vi "TestExec.Result Option, Level to Control.vi"(10 "Level":i32) -> (2 "Result Sel Out":T1=1 items=["Enabled", "Disabled"])   [LabVIEW 2018]
uses:
  TestExec.Result Option Selector.ctl
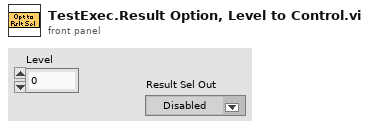
[diagram p1: front panel]
types:
  T1 = typedef "TestExec.Result Option Selector.ctl" = u16
  T2 = cluster{"Color":u32, "Factory Logix":bool, "Data Whs":bool}
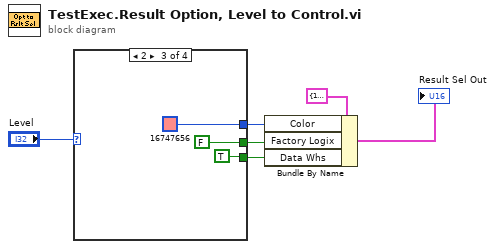
[diagram p0: block diagram]
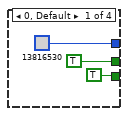
[diagram p2: hidden frame]
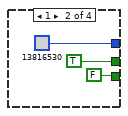
[diagram p3: hidden frame]
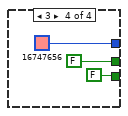
[diagram p4: hidden frame]
diagram:
  n1 = case shown="2" "Level" {
    tunnel: [u32 13816530 u32 13816530 u32 16747656 u32 16747656] -> w3
    tunnel: [TRUE TRUE FALSE FALSE] -> w2
    tunnel: [TRUE FALSE TRUE FALSE] -> w1
    frame 0, Default {
    }
    frame 1 {
    }
    frame 2 {
    }
    frame 3 {
    }
  }
  n2 = Bundle By Name(cluster=T2 {"Color"=13816530, "Factory Logix"=TRUE, "Data Whs"=TRUE} ("Result Sel Out"), "Color"=w3, "Factory Logix"=w2, "Data Whs"=w1) -> (→"Result Sel Out":T2)
